vi "WFGConfigureReadBack.vi"(0 "object in":refnum<class "AD2_WFG_SDK.lvclass">, 2 "Ch":T1={"idxChannel"=0, "Settings out of range"=FALSE, "Carrier"={"Frequency (Hz)"=1000.0, "Amplitude (V)"=1.0, "Offset(V)"=0.0, "Symmetry(%) "=50.0, "Phase(Deg)"=0.0, "Function"=1, "Enable"=FALSE}, "Trigger"={"secRun(0=Cont)"=0.0, "secWait"=0.0, "cRepeat(0=inf)"=0, "Repeat Trigger"=FALSE, "TrigrSrc"=enum."trigrsrcNone"}, "FM Mod"={"Frequency (Hz)"=1000.0, "Amplitude (%)"=1.0, "Offset(V)"=0.0, "Symmetry(%) "=50.0, "Phase(Deg)"=0.0, "Function 2"=1, "Enable"=FALSE}} {"FM Mod"."Function 2" items=["DC"=0, "Sine"=1, "Square"=2, "Triangle"=3, "RampUp"=4, "RampDown"=5, "Noise"=6, "Pulse"=7, "Custom"=30]; "Carrier"."Function" items=["DC"=0, "Sine"=1, "Square"=2, "Triangle"=3, "RampUp"=4, "RampDown"=5, "Noise"=6, "Pulse"=7, "Custom"=30]}, 5 "error in (no error)":errorcluster) -> (14 "object out":refnum<class "AD2_WFG_SDK.lvclass">, 16 "Ch out":T1={"idxChannel"=0, "Settings out of range"=FALSE, "Carrier"={"Frequency (Hz)"=1000.0, "Amplitude (V)"=1.0, "Offset(V)"=0.0, "Symmetry(%) "=50.0, "Phase(Deg)"=0.0, "Function"=1, "Enable"=FALSE}, "Trigger"={"secRun(0=Cont)"=0.0, "secWait"=0.0, "cRepeat(0=inf)"=0, "Repeat Trigger"=FALSE, "TrigrSrc"=enum."trigrsrcNone"}, "FM Mod"={"Frequency (Hz)"=1000.0, "Amplitude (%)"=1.0, "Offset(V)"=0.0, "Symmetry(%) "=50.0, "Phase(Deg)"=0.0, "Function 2"=1, "Enable"=FALSE}} {"FM Mod"."Function 2" items=["DC"=0, "Sine"=1, "Square"=2, "Triangle"=3, "RampUp"=4, "RampDown"=5, "Noise"=6, "Pulse"=7, "Custom"=30]; "Carrier"."Function" items=["DC"=0, "Sine"=1, "Square"=2, "Triangle"=3, "RampUp"=4, "RampDown"=5, "Noise"=6, "Pulse"=7, "Custom"=30]}, 19 "error out":errorcluster)   [LabVIEW 2019, in "AD2_WFG_SDK.lvclass"]
uses:
  AD2_WFG_SDK.lvclass
  WFGCh.ctl
  AD2TriggerSources.ctl
  AD2_WFG_SDK.lvclass/AD2_WFG_SDK.ctl
  Olasdwf/Olasdwf.lvlib
  AD2_SDK_class/AD2_SDK.lvclass
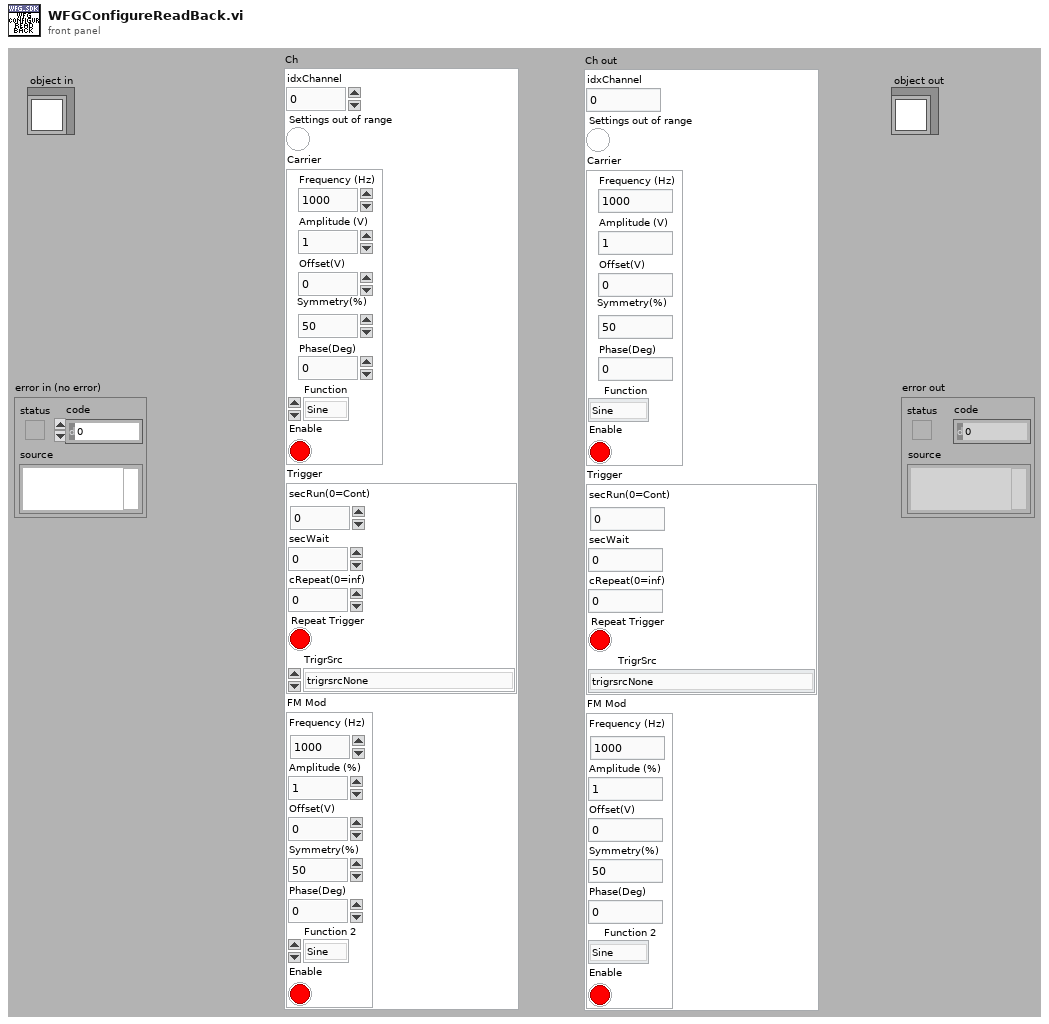
[diagram p1: front panel]
types:
  T1 = typedef "AD2_WFG_SDK.lvclass/WFGCh.ctl" = cluster{"idxChannel":i32, "Settings out of range":bool, "Carrier":cluster{"Frequency (Hz)":dbl, "Amplitude (V)":dbl, "Offset(V)":dbl, "Symmetry(%) ":dbl, "Phase(Deg)":dbl, "Function":u16, "Enable":bool}, "Trigger":cluster{"secRun(0=Cont)":dbl, "secWait":dbl, "cRepeat(0=inf)":i32, "Repeat Trigger":bool, "TrigrSrc":T2}, "FM Mod":cluster{"Frequency (Hz)":dbl, "Amplitude (%)":dbl, "Offset(V)":dbl, "Symmetry(%) ":dbl, "Phase(Deg)":dbl, "Function 2":u16, "Enable":bool}}
  T2 = typedef "AD2_SDK.lvclass/AD2TriggerSources.ctl" = enum8{"trigrsrcNone", "trigsrcPC", "trigsrcDetectorAnalogIn", "trigsrcDetectorDigitalIn", "trigsrcAnalogIn", "trigsrcDigitalIn", "trigsrcDigitalOut", "trigsrcAnalogOut1", "trigsrcAnalogOut2", "trigsrcAnalogOut3", "trigsrcAnalogOut4", "trigsrcExternal1", "trigsrcExternal2", "trigsrcExternal3", "trigsrcExternal4", ""}
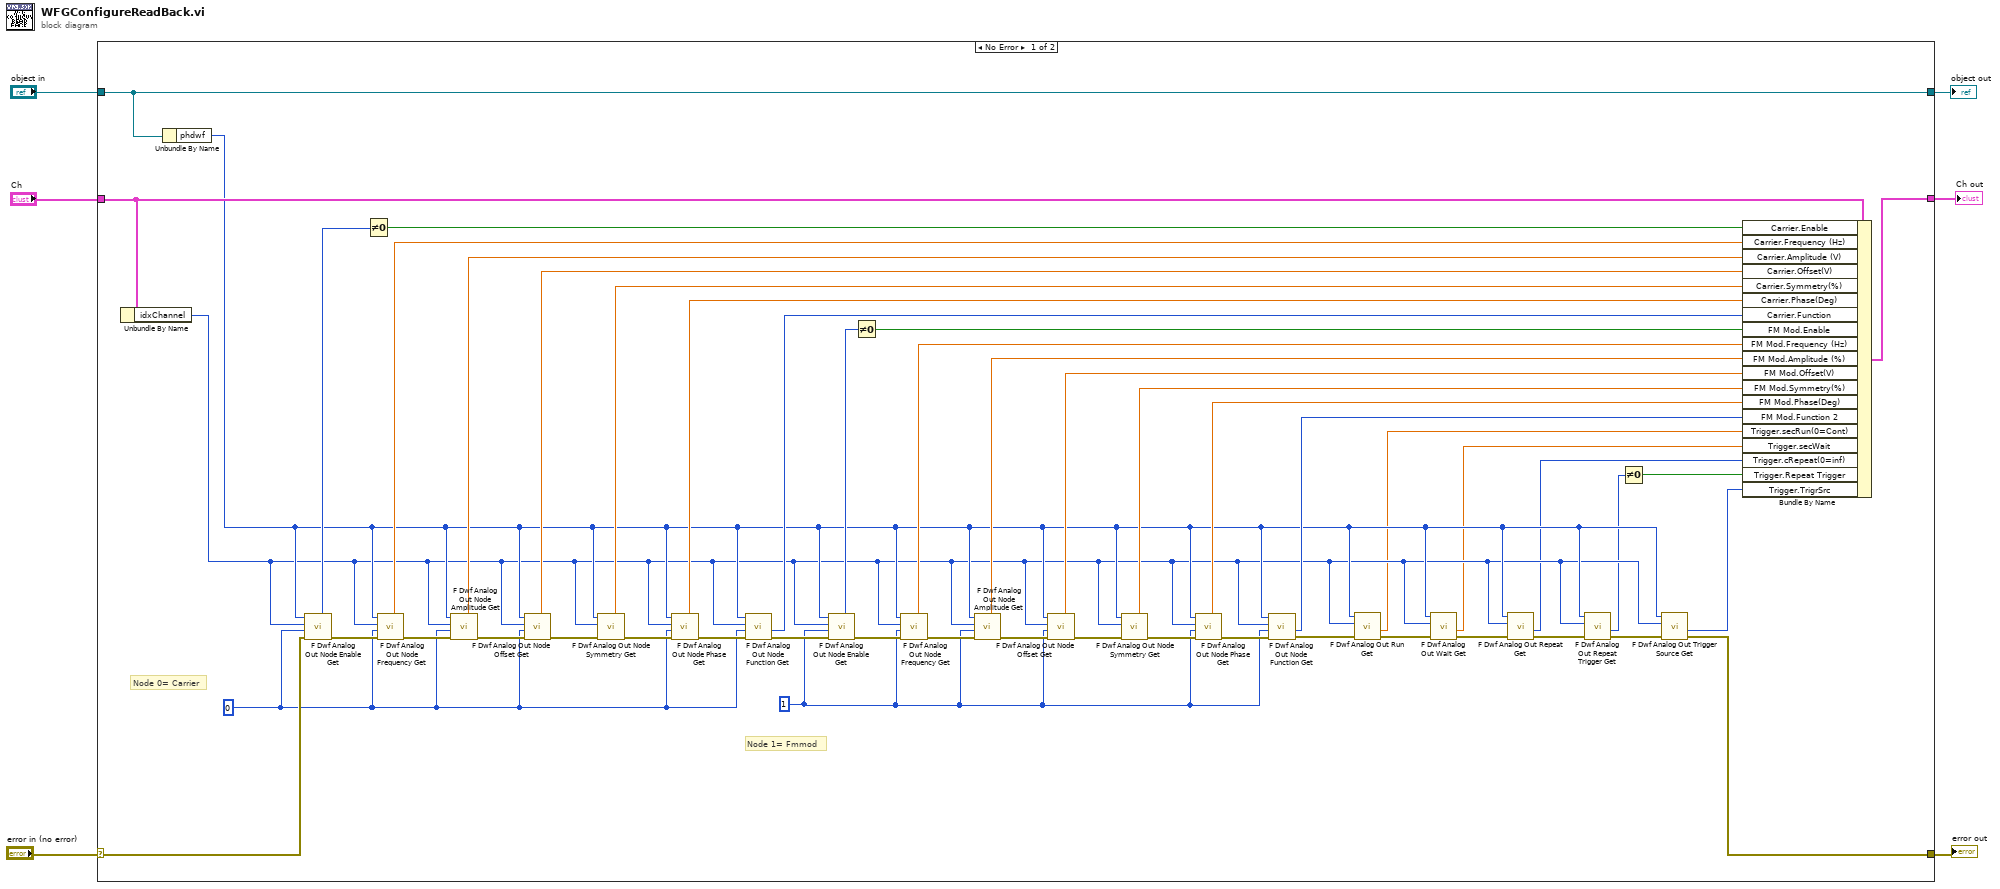
[diagram p0: block diagram]
diagram:
  n1 = case shown="No Error" "error in (no error)" {
    selector: "error in (no error)" -> [w39 w57]
    tunnel: [w7 w57] -> w5
    tunnel: [w55 w56] -> w3
    tunnel: "object in" -> [w55 w56]
    tunnel: "Ch" -> [w40 _]
    tunnel: [w38 _] -> w1
    frame No Error {
      w29 = 1 ("node")
      w37 = 0 ("node")
      # "Node 1= Fmmod"
      # "Node 0= Carrier"
      n2 = Unbundle By Name(w40) -> ("idxChannel"=w15:i32)
      n3 = Unbundle By Name(w55) -> ("phdwf"=w16:i32)
      n4 = call "F Dwf Analog Out Node Enable Get.vi"("error in (no error)"=w39, "node"=w37, "idxChannel"=w15, "hdwf"=w16) -> ("error out"=w41:errorcluster, "pfEnable out"=w47:i32)  [unwired: 5 in, 1 out]
      n5 = Not Equal To 0?(x=w47) -> (x != 0?=w46:bool)
      n6 = call "F Dwf Analog Out Node Frequency Get.vi"("error in (no error)"=w41, "node"=w37, "idxChannel"=w15, "hdwf"=w16) -> ("error out"=w42:errorcluster, "phzFrequency out"=w48:dbl)  [unwired: 5 in, 1 out]
      n7 = call "F Dwf Analog Out Node Amplitude Get.vi"("error in (no error)"=w42, "node"=w37, "idxChannel"=w15, "hdwf"=w16) -> ("error out"=w43:errorcluster, "pvAmplitude out"=w49:dbl)  [unwired: 5 in, 1 out]
      n8 = call "F Dwf Analog Out Node Offset Get.vi"("error in (no error)"=w43, "node"=w37, "idxChannel"=w15, "hdwf"=w16) -> ("error out"=w44:errorcluster, "pvOffset out"=w50:dbl)  [unwired: 5 in, 1 out]
      n9 = call "F Dwf Analog Out Node Symmetry Get.vi"("error in (no error)"=w44, "idxChannel"=w15, "hdwf"=w16) -> ("error out"=w45:errorcluster, "ppercentageSymmetry out"=w51:dbl)  [unwired: 6 in, 1 out]
      n10 = call "F Dwf Analog Out Node Phase Get.vi"("error in (no error)"=w45, "node"=w37, "idxChannel"=w15, "hdwf"=w16) -> ("error out"=w52:errorcluster, "pdegreePhase out"=w54:dbl)  [unwired: 5 in, 1 out]
      n11 = call "F Dwf Analog Out Node Function Get.vi"("error in (no error)"=w52, "node"=w37, "idxChannel"=w15, "hdwf"=w16) -> ("error out"=w30:errorcluster, "pfunc"=w53:u8)  [unwired: 5 in, 1 out]
      n12 = call "F Dwf Analog Out Node Enable Get.vi"("error in (no error)"=w30, "node"=w29, "idxChannel"=w15, "hdwf"=w16) -> ("error out"=w31:errorcluster, "pfEnable out"=w28:i32)  [unwired: 5 in, 1 out]
      n13 = Not Equal To 0?(x=w28) -> (x != 0?=w27:bool)
      n14 = call "F Dwf Analog Out Node Frequency Get.vi"("error in (no error)"=w31, "node"=w29, "idxChannel"=w15, "hdwf"=w16) -> ("error out"=w32:errorcluster, "phzFrequency out"=w26:dbl)  [unwired: 5 in, 1 out]
      n15 = call "F Dwf Analog Out Node Amplitude Get.vi"("error in (no error)"=w32, "node"=w29, "idxChannel"=w15, "hdwf"=w16) -> ("error out"=w33:errorcluster, "pvAmplitude out"=w25:dbl)  [unwired: 5 in, 1 out]
      n16 = call "F Dwf Analog Out Node Offset Get.vi"("error in (no error)"=w33, "node"=w29, "idxChannel"=w15, "hdwf"=w16) -> ("error out"=w34:errorcluster, "pvOffset out"=w24:dbl)  [unwired: 5 in, 1 out]
      n17 = call "F Dwf Analog Out Node Symmetry Get.vi"("error in (no error)"=w34, "idxChannel"=w15, "hdwf"=w16) -> ("error out"=w35:errorcluster, "ppercentageSymmetry out"=w23:dbl)  [unwired: 6 in, 1 out]
      n18 = call "F Dwf Analog Out Node Phase Get.vi"("error in (no error)"=w35, "node"=w29, "idxChannel"=w15, "hdwf"=w16) -> ("error out"=w36:errorcluster, "pdegreePhase out"=w22:dbl)  [unwired: 5 in, 1 out]
      n19 = call "F Dwf Analog Out Node Function Get.vi"("error in (no error)"=w36, "node"=w29, "idxChannel"=w15, "hdwf"=w16) -> ("error out"=w8:errorcluster, "pfunc"=w21:u8)  [unwired: 5 in, 1 out]
      n20 = call "F Dwf Analog Out Run Get.vi"("error in (no error)"=w8, "idxChannel"=w15, "hdwf"=w16) -> ("error out"=w20:errorcluster, "psecRun out"=w14:dbl)  [unwired: 6 in, 1 out]
      n21 = call "F Dwf Analog Out Wait Get.vi"("error in (no error)"=w20, "idxChannel"=w15, "hdwf"=w16) -> ("error out"=w19:errorcluster, "psecWait out"=w13:dbl)  [unwired: 6 in, 1 out]
      n22 = call "F Dwf Analog Out Repeat Get.vi"("error in (no error)"=w19, "idxChannel"=w15, "hdwf"=w16) -> ("error out"=w18:errorcluster, "pcRepeat out"=w12:i32)  [unwired: 6 in, 1 out]
      n23 = call "F Dwf Analog Out Repeat Trigger Get.vi"("error in (no error)"=w18, "idxChannel"=w15, "hdwf"=w16) -> ("error out"=w17:errorcluster, "pfRepeatTrigger out"=w11:i32)  [unwired: 6 in, 1 out]
      n24 = Not Equal To 0?(x=w11) -> (x != 0?=w10:bool)
      n25 = call "F Dwf Analog Out Trigger Source Get.vi"("error in (no error)"=w17, "idxChannel"=w15, "hdwf"=w16) -> ("error out"=w7:errorcluster, "ptrigsrc"=w9:u8)  [unwired: 6 in, 1 out]
      n26 = Bundle By Name(cluster=w40, "Carrier.Enable"=w46, "Carrier.Frequency (Hz)"=w48, "Carrier.Amplitude (V)"=w49, "Carrier.Offset(V)"=w50, "Carrier.Symmetry(%)"=w51, "Carrier.Phase(Deg)"=w54, "Carrier.Function"=w53, "FM Mod.Enable"=w27, "FM Mod.Frequency (Hz)"=w26, "FM Mod.Amplitude (%)"=w25, "FM Mod.Offset(V)"=w24, "FM Mod.Symmetry(%)"=w23, "FM Mod.Phase(Deg)"=w22, "FM Mod.Function 2"=w21, "Trigger.secRun(0=Cont)"=w14, "Trigger.secWait"=w13, "Trigger.cRepeat(0=inf)"=w12, "Trigger.Repeat Trigger"=w10, "Trigger.TrigrSrc"=w9) -> (w38:T1)
    }
    frame Error {
    }
  }
  "error out" <- w5
  "object out" <- w3
  "Ch out" <- w1
